vi "Function.vi"(8 "error in":errorcluster, 11 "reference":refnum<vi>) -> (0 "error out":errorcluster, 3 "Function out":refnum<class "Function.lvclass">)   [LabVIEW 2014, in "Raspberry Pi Compatible Compiler for LabVIEW.lvlib" / "Function.lvclass"]
uses:
  Function.lvclass
  Node/Node.lvclass
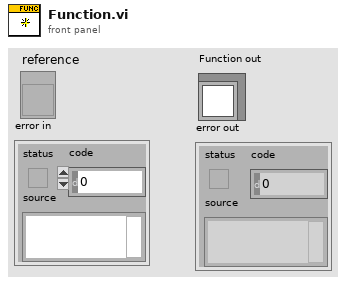
[diagram p1: front panel]
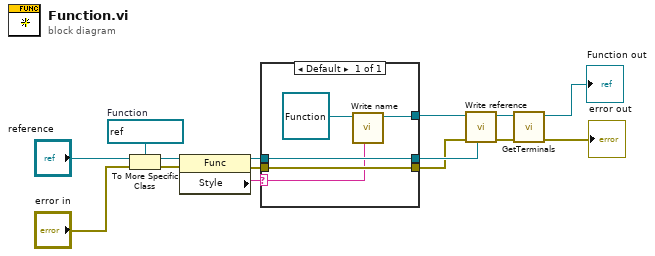
[diagram p0: block diagram]
diagram:
  w15 = refnum<vi> refnum  # Function
  n1 = To More Specific Class(target class=w15, reference="reference", error in="error in") -> (specific class reference=w12:refnum<vi>, error out=w11:errorcluster)
  n2 = property class="Func"(reference=w12, error in=w11) -> (reference out=w3:refnum<vi>, error out=w4:errorcluster, "Style"=w5:string)
  n3 = case shown="Default" w5 {
    selector: w5 -> [w17]
    tunnel: [w18] -> w10
    tunnel: w3 -> [w20]
    tunnel: [w20] -> w9
    tunnel: w4 -> [w19]
    tunnel: [w19] -> w8
    frame Default {
      n4 = call-dynamic "Write name.vi"("name"=w17, "Node in"=refnum<class "Function.lvclass"> refnum ("Function in")) -> ("Node out"=w18:refnum<class "Function.lvclass">)  [unwired: 7 in]
    }
  }
  n5 = call-dynamic "Write reference.vi"("reference"=w9, "error in"=w8, "GObject in"=w10) -> ("error out"=w6:errorcluster, "GObject out"=w7:refnum<class "Function.lvclass">)  [unwired: 5 in]
  n6 = call "GetTerminals.vi"("error in"=w6, "Node in"=w7) -> ("error out"=→"error out":errorcluster, "Node out"=→"Function out":refnum<class "Function.lvclass">)  [unwired: 8 in]
